vi "SetDefaultPipleline.vi"(8 "error in (no error)":errorcluster, 10 "Image Pipleline In":refnum<class "ImagePipeline.lvclass">, 11 "Microscope in":refnum<class "Microscope.lvclass">) -> (0 "error out":errorcluster, 3 "Microscope out":refnum<class "Microscope.lvclass">)   [LabVIEW 2020, in "Microscope.lvlib" / "Microscope.lvclass"]
uses:
  Microscope.lvclass
  C:/Program Files/National Instruments/LabVIEW 2020/vi.lib/ActorFramework/Actor/Actor.lvclass
  ImagePipeline/ImagePipeline.lvclass
  Microscope.lvclass/Microscope.ctl
  <vilib>/ActorFramework/Actor/Actor.lvclass
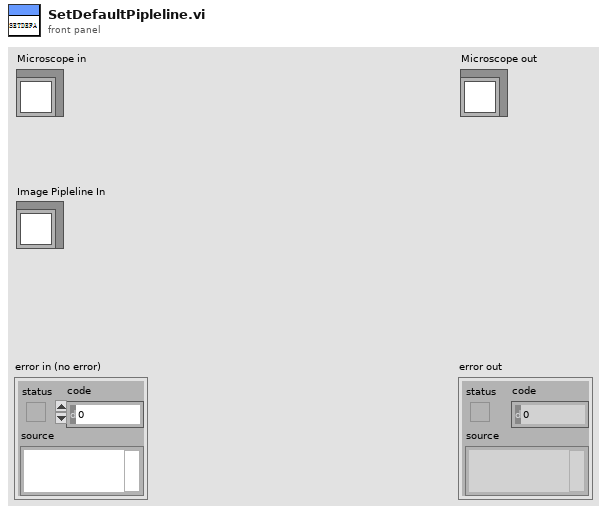
[diagram p1: front panel]
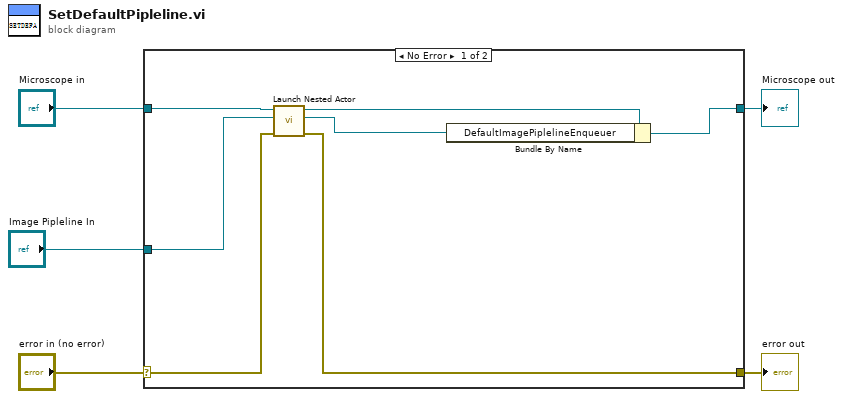
[diagram p0: block diagram]
diagram:
  n1 = case shown="No Error" "error in (no error)" {
    selector: "error in (no error)" -> [w9 w14]
    tunnel: [w8 w14] -> w4
    tunnel: [w12 w13] -> w2
    tunnel: "Microscope in" -> [w11 w13]
    tunnel: "Image Pipleline In" -> [w10 _]
    frame No Error {
      n2 = call <vilib>:"Launch Nested Actor.vi"("error in (no error)"=w9, "Nested Actor"=w10, "Caller Actor in"=w11) -> ("error out"=w8:errorcluster, "Nested Actor's Enqueuer"=w6:refnum<class "Message Enqueuer.lvclass">, "Caller Actor out"=w7:refnum<class "Microscope.lvclass">)  [unwired: 6 in]
      n3 = Bundle By Name(cluster=w7, "DefaultImagePiplelineEnqueuer"=w6) -> (w12:refnum<class "Microscope.lvclass">)
    }
    frame Error {
    }
  }
  "error out" <- w4
  "Microscope out" <- w2
